vi "Read modbus channels.vi"(8 "error in":errorcluster, 11 "Modbus Slave configuration in":refnum<class "Modbus Slave configuration.lvclass">) -> (0 "error out":errorcluster, 2 "modbus channels":refnum<class "Modbus Module Channel.lvclass">[](array[class]), 3 "Modbus Slave configuration out":refnum<class "Modbus Slave configuration.lvclass">)   [LabVIEW 2013, in "Modbus Slave configuration.lvclass"]
uses:
  Modbus Slave configuration.lvclass
  module channel/Modbus Module Channel.lvclass
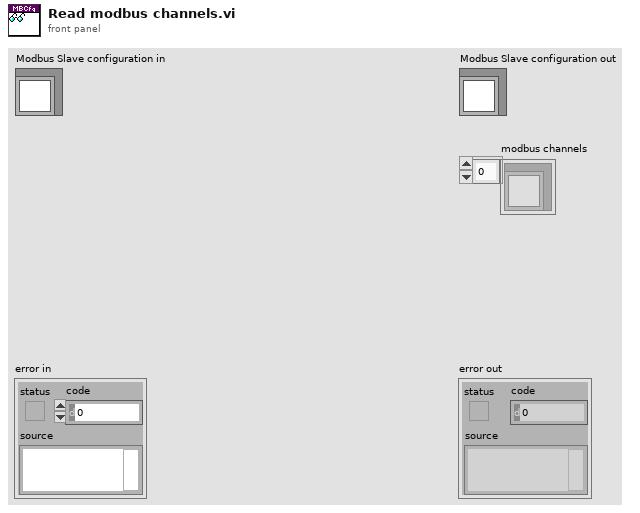
[diagram p1: front panel]
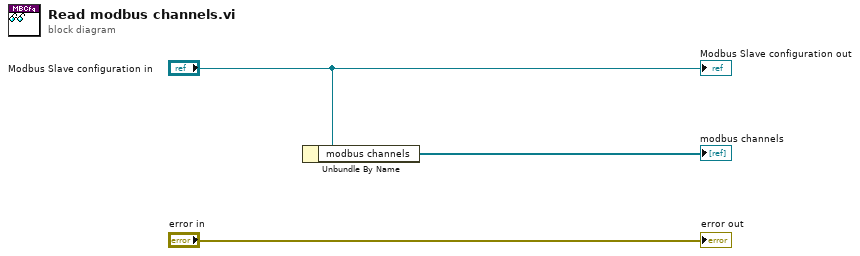
[diagram p0: block diagram]
diagram:
  n1 = Unbundle By Name("Modbus Slave configuration in") -> ("modbus channels"=→"modbus channels":refnum<class "Modbus Module Channel.lvclass">[])
  "error out" <- "error in"
  "Modbus Slave configuration out" <- "Modbus Slave configuration in"
